vi "Close IO Trace.vi"(8 "error in (no error)":errorcluster) -> (0 "error out":errorcluster)   [LabVIEW 2010, in "NI IO Trace.lvlib"]
doc: "This VI closes NI I/O Trace. To start logging again, restart NI I/O Trace."
uses:
  <vilib>/NiIOTrace/NI IO Trace.lvlib
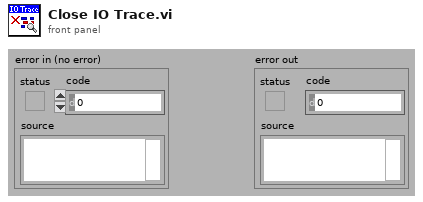
[diagram p1: front panel]
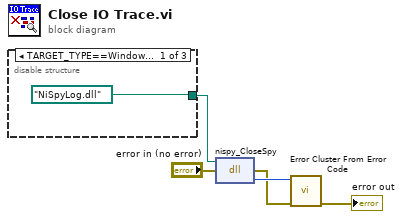
[diagram p0: block diagram]
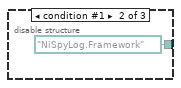
[diagram p2: hidden frame]
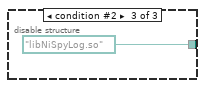
[diagram p3: hidden frame]
diagram:
  n1 = disable-structure shown="TARGET_TYPE==Windows, default" {
    disable-tunnel: [path "NiSpyLog.dll" ("path in") path "NiSpyLog.Framework" ("path in") path "libNiSpyLog.so" ("path in")] -> w3
    frame condition #0 (active) {
    }
    frame condition #1 {
    }
    frame condition #2 {
    }
  }
  n2 = dll-call lib="C:/WINDOWS/system32/NiSpyLog.dll" fn="nispy_CloseSpy"(path in=w3, error in="error in (no error)") -> (error out=w2:errorcluster, "return type"=w4:i32)  [unwired: 1 in, 1 out]
  n3 = call <vilib>:"Error Cluster From Error Code.vi"("error in (no error)"=w2, "error code (0)"=w4) -> ("error out"=→"error out":errorcluster)  [unwired: 1 in, 6 out]
